vi "Stop Test.vi"(8 "error in (no error)":errorcluster, 11 "Coverage Report in":refnum<class "Coverage Report.lvclass">) -> (0 "error out":errorcluster, 3 "Coverage Report out":refnum<class "Coverage Report.lvclass">)   [LabVIEW 2020, in "Coverage Report.lvclass"]
uses:
  Coverage Report.lvclass
  Coverage Report.lvclass/Coverage Report.ctl
  <vilib>/Platform/browser.llb/Open URL in Default Browser (path).vi
  c80752a9-34a8-4590-82a2-f6539b8745c6.vi
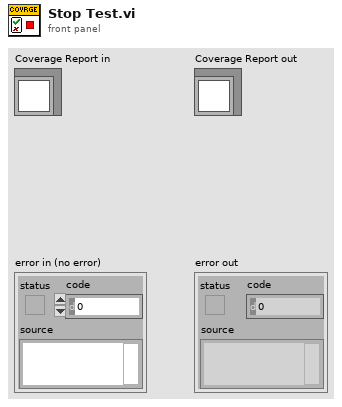
[diagram p1: front panel]
types:
  T1 = enum16{"open", "replace", "create", "open or create", "replace or create", "replace or create with confirmation"}
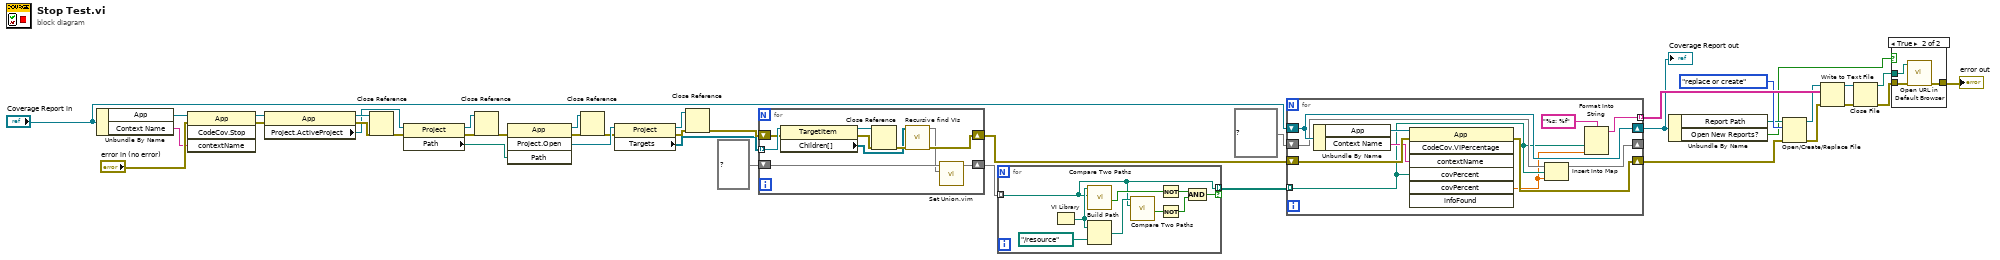
[diagram p0: block diagram]
diagram:
  n1 = Unbundle By Name("Coverage Report in") -> ("App"=w2:refnum<vi>, "Context Name"=w3:string)
  n2 = invoke class="App" method="CodeCov.Stop"(reference=w2, error in="error in (no error)", "contextName"=w3) -> (reference out=w10:refnum<vi>, error out=w13:errorcluster)  [unwired: 1 in, 2 out]
  n3 = property class="App"(reference=w10, error in=w13) -> (reference out=w5:refnum<vi>, error out=w8:errorcluster, "Project.ActiveProject"=w4:refnum<vi>)
  n4 = Close Reference(reference=w5, error in (no error)=w8) -> (error out=w9:errorcluster)
  n5 = property class="Project"(reference=w4, error in=w9) -> (reference out=w6:refnum<vi>, error out=w7:errorcluster, "Path"=w12:path)
  n6 = Close Reference(reference=w6, error in (no error)=w7) -> (error out=w14:errorcluster)
  n7 = invoke class="App" method="Project.Open"(error in=w14, "Path"=w12) -> (reference out=w19:refnum<vi>, error out=w23:errorcluster, "Project:Open"=w25:refnum<vi>)  [unwired: 2 in, 1 out]
  n8 = Close Reference(reference=w19, error in (no error)=w23) -> (error out=w20:errorcluster)
  n9 = property class="Project"(reference=w25, error in=w20) -> (reference out=w21:refnum<vi>, error out=w24:errorcluster, "Targets"=w16:refnum<vi>[])
  n10 = Close Reference(reference=w21, error in (no error)=w24) -> (error out=w22:errorcluster)
  n11 = for {
    tunnel: w16 -> [w50] mode=indexing
    shift-right: [w47] -> w11
    shift-left: w22 -> [w48]
    shift-right: [w43] -> w17
    shift-left: set{path} {} ("VIs") -> [w45]
    n12 = property class="TargetItem"(reference=w50, error in=w48) -> (reference out=w46:refnum<vi>, error out=w49:errorcluster, "Children[]"=w41:refnum<vi>[])
    n13 = Close Reference(reference=w46, error in (no error)=w49) -> (error out=w42:errorcluster)
    n14 = call "Recursive find VIs.vi"("error in (no error)"=w42, "Project Items"=w41) -> ("error out"=w47:errorcluster, "VIs"=w44:set{path})  [unwired: 8 in]
    n15 = call "Set Union.vim"("set 2"=w44, "set 1"=w45) -> ("union"=w43:set{path})  [unwired: 9 in]
  }
  n16 = for {
    tunnel: w17 -> [w51] mode=indexing
    tunnel: [w51] -> w26 mode=indexing if=w56
    n17 = VI Library() -> (path=w54:path)
    n18 = call <vilib>:"Compare Two Paths.vi"("Path 2"=w51, "Path 1"=w54) -> ("Path 2 Relative to Path 1?"=w59:bool)  [unwired: 6 in, 3 out]
    n19 = Build Path(base path=w54, name or relative path=path "../resource") -> (appended path=w52:path)
    n20 = call <vilib>:"Compare Two Paths.vi"("Path 2"=w51, "Path 1"=w52) -> ("Path 2 Relative to Path 1?"=w57:bool)  [unwired: 6 in, 3 out]
    n21 = Not(x=w59) -> (.not. x?=w58:bool)
    n22 = Not(x=w57) -> (.not. x?=w55:bool)
    n23 = And(x=w58, y=w55) -> (x .and. y?=w56:bool)
  }
  n24 = for {
    shift-right: [w70] -> w1
    shift-left: "Coverage Report in" -> [w70]
    shift-right: [w68] -> w34
    shift-left: w11 -> [w69]
    tunnel: w26 -> [w62] mode=indexing
    shift-right: [w66] -> _
    shift-left: map{path, dbl} {} ("Code Coverage") -> [w67]
    tunnel: [w60] -> w36 mode=indexing
    n25 = Unbundle By Name(w70) -> ("App"=w64:refnum<vi>, "Context Name"=w65:string)
    n26 = invoke class="App" method="CodeCov.VIPercentage"(reference=w64, error in=w69, "contextName"=w65, "covPercent"=w62) -> (error out=w68:errorcluster, "covPercent"=w61:dbl)  [unwired: 3 in, 5 out]
    n27 = Insert Into Map(map in=w67, key=w62, value=w61) -> (map out=w66:map{path, dbl})  [unwired: 2 out]
    n28 = Format Into String(format string="%s: %f", w62, w61) -> (resulting string=w60:string)  [unwired: 2 in, 1 out]
  }
  "Coverage Report out" <- w1
  n29 = Unbundle By Name(w1) -> ("Report Path"=w32:path, "Open New Reports?"=w27:bool)
  n30 = Open/Create/Replace File(file path (use dialog)=w32, error in=w34, operation (0:open)=T1."replace or create") -> (refnum out=w28:refnum<file>, error out=w29:errorcluster)  [unwired: 3 in, 1 out]
  n31 = Write to Text File(file (use dialog)=w28, text=w36, error in=w29) -> (refnum out=w30:refnum<file>, error out=w31:errorcluster)  [unwired: 1 in, 1 out]
  n32 = Close File(refnum=w30, error in=w31) -> (path=w39:path, error out=w33:errorcluster)
  n33 = case shown="True" w27 {
    tunnel: w39 -> [_ w72]
    tunnel: w33 -> [w71 w74]
    tunnel: [w71 w73] -> w37
    frame False {
    }
    frame True {
      n34 = call-poly <vilib>:"Open URL in Default Browser.vi"("error in (no error)"=w74, "path"=w72) -> ("error out"=w73:errorcluster)  [unwired: 4 in, 1 out]
    }
  }
  "error out" <- w37
